vi "Activate Redline.vi"(8 "error in (no error)":errorcluster, 10 "Redline Index":i32, 11 "DataProcessor in":refnum<class "DataProcessor.lvclass">) -> (0 "error out":errorcluster, 3 "DataProcessor out":refnum<class "DataProcessor.lvclass">)   [LabVIEW 2020, in "Volatus.lvlib" / "DataProcessor.lvclass"]
uses:
  DataProcessor.lvclass
  DataProcessor.lvclass/DataProcessor.ctl
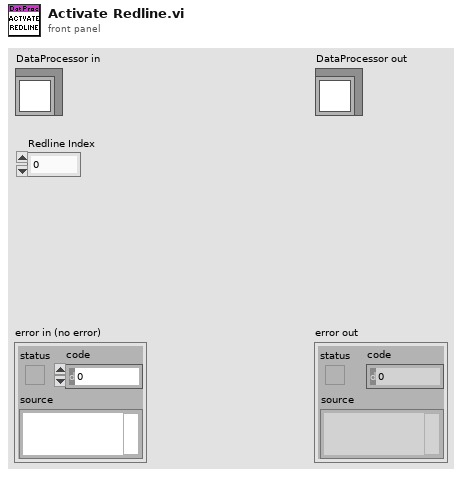
[diagram p1: front panel]
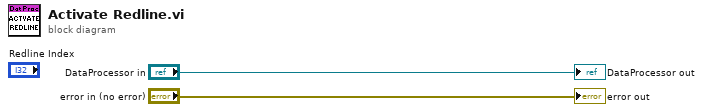
[diagram p0: block diagram]
diagram:
  "error out" <- "error in (no error)"
  "DataProcessor out" <- "DataProcessor in"
